vi "Day 1 Task 1.vi"() -> ()   [LabVIEW 2018]
panel:
  out "sum":i16
  out "array w/ subset deleted":bool[](array[boolean])
  out "Log":string[](array[string])
  out "Array":bool[](array[boolean])
  out "Sea floor depths":i32[](array[numeric])
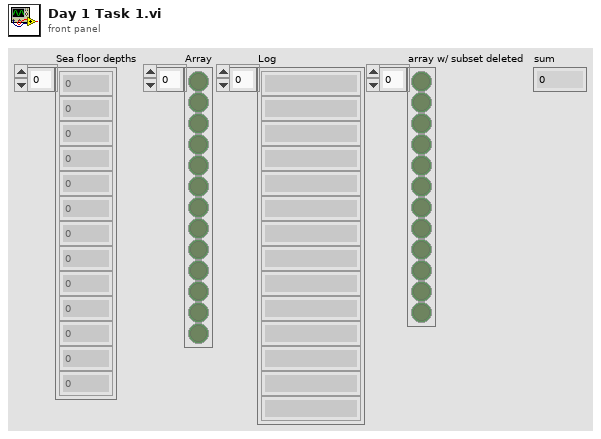
[diagram p1: front panel]
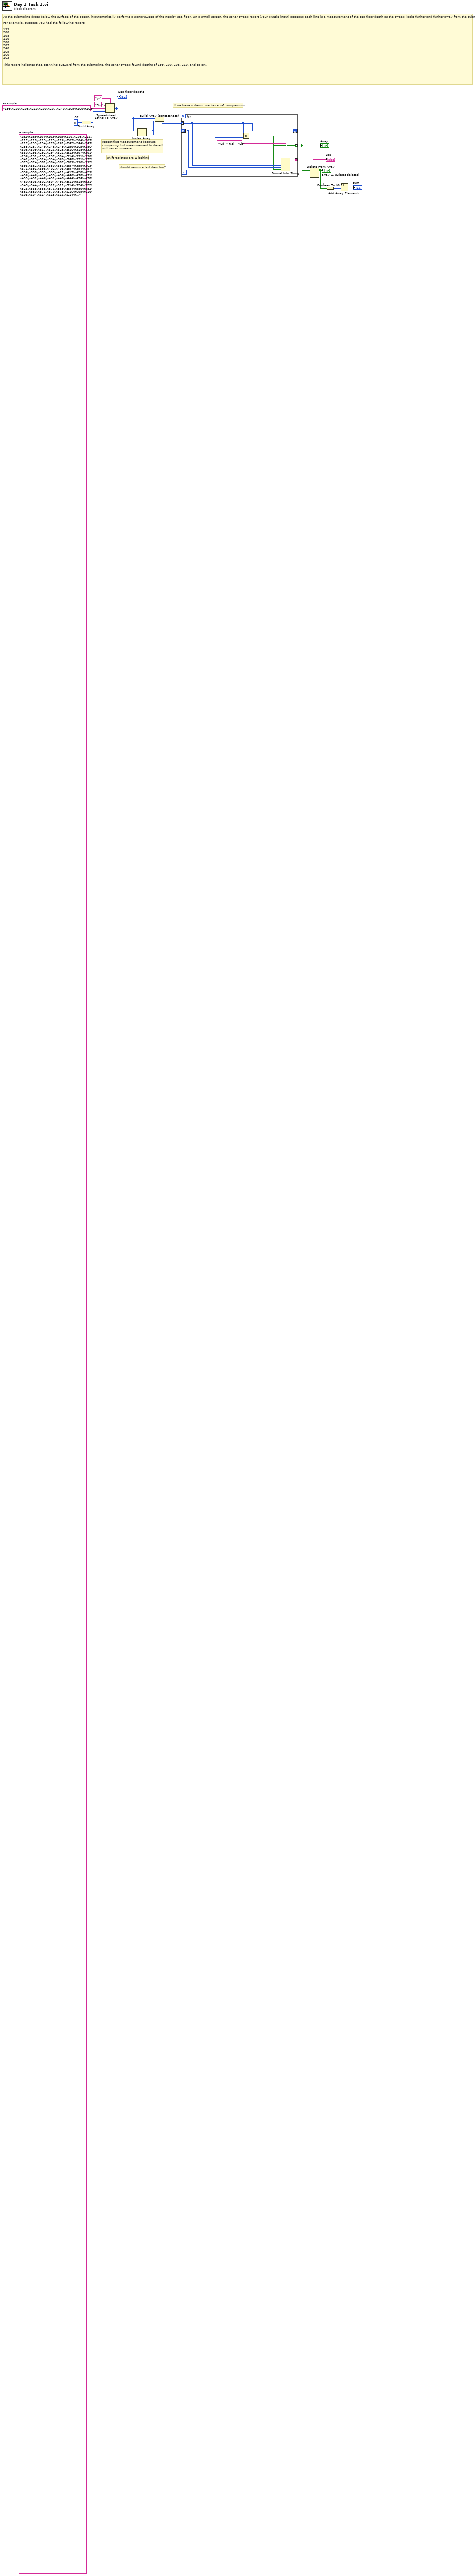
[diagram p0: block diagram]
diagram:
  w1 = "182\n188\n204\n203\n205\n206\n208\n216\n217\n218\n219\n225\n226\n207\n204\n205\n217\n255\n254\n270\n261\n262\n264\n265\n255\n257\n249\n248\n249\n250\n265\n286\n308\n309\n317\n326\n328\n316\n318\n333\n330\n293\n292\n294\n321\n313\n307\n301\n296\n291\n295\n297\n304\n314\n331\n330\n342\n325\n324\n354\n360\n368\n371\n372\n373\n374\n381\n384\n387\n389\n390\n392\n393\n382\n361\n350\n356\n357\n359\n363\n371\n391\n398\n402\n403\n397\n394\n397\n396\n398\n399\n393\n411\n417\n428\n429\n456\n446\n451\n459\n456\n460\n458\n451\n455\n452\n446\n451\n448\n444\n476\n478\n480\n503\n502\n504\n496\n511\n518\n531\n543\n544\n516\n512\n511\n514\n524\n522\n523\n535\n558\n576\n589\n584\n580\n582\n581\n580\n571\n570\n578\n616\n609\n610\n603\n604\n614\n615\n616\n614\n..."  # example
  w10 = 0  # i32
  (unwired) "199\n200\n208\n210\n200\n207\n240\n269\n260\n263"  # example
  # "shift registers are 1 behind"
  # "should remove last item too?"
  # "If we have n items, we have n-1 comparisons"
  # "repeat first measurement because\ncomparing first measurement to iteself\nwill never increase"
  # "As the submarine drops below the surface of the ocean, it automatically performs a sonar sweep of the nearby sea floor. On a small screen, the sonar sweep report (your puzzle input) appears: each line is a measurement of the sea floor depth as the sweep looks further and further away from the submarine.\n\nFor example, suppose you had the following report:\n\n199\n200\n208\n210\n200\n207\n240\n269\n260\n263\n\nThis report indicates that, scanning outward from the submarine, the sonar sweep found depths of 199, 200, 208, 210, and so on."
  n1 = Build Array(w10) -> (w11:i32[])
  n2 = Spreadsheet String To Array(delimiter (Tab)="\n", format string="%d", spreadsheet string=w1, array type (2D Dbl)=w11) -> (array=w9:i32[])
  "Sea floor depths" <- w9
  n3 = Index Array(array=w9) -> (element=w7:i32)  [unwired: 1 in]
  n4 = Build Array (concatenate)(w9, w7) -> (w8:i32[])
  n5 = for {
    tunnel: w8 -> [w17] mode=indexing
    shift-right: [w17] -> _
    shift-left: w7 -> [w16]
    tunnel: [w15] -> w5 mode=indexing
    tunnel: [w14] -> w6 mode=indexing
    n6 = Greater?(x=w17, y=w16) -> (0:w15:bool)
    n7 = Format Into String(format string="%d > %d = %b", w17, w16, w15) -> (resulting string=w14:string)  [unwired: 2 in, 1 out]
  }
  "Array" <- w5
  "Log" <- w6
  n8 = Delete From Array(array=w5) -> (array with subset deleted=w4:bool[])  [unwired: 2 in, 1 out]
  "array w/ subset deleted" <- w4
  n9 = Boolean To (0,1)(Boolean=w4) -> (0, 1=w3:i16[])
  n10 = Add Array Elements(numeric array=w3) -> (sum=→"sum":i16)
